vi "Build Log Path.vi"(11 "Project Path":path) -> (0 "error out":errorcluster, 3 "PantherLAB Log File Path":path)   [LabVIEW 2016, in "PantherLAB_Scripting.lvlib"]
uses:
  PantherLAB_Scripting.lvlib
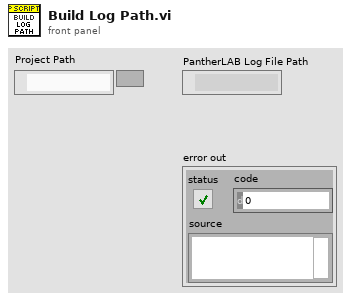
[diagram p1: front panel]
types:
  T1 = enum16{"open", "replace", "create", "open or create", "replace or create", "replace or create with confirmation"}
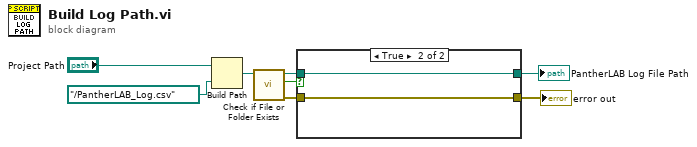
[diagram p0: block diagram]
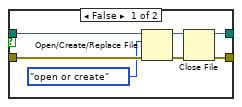
[diagram p2: hidden frame]
diagram:
  n1 = Build Path(base path="Project Path", name or relative path=path "../PantherLAB_Log.csv") -> (appended path=w4:path)
  n2 = call <vilib>:"Check if File or Folder Exists.vi"("path"=w4) -> ("error out"=w8:errorcluster, "file or folder exists?"=w3:bool, "dup path"=w2:path)  [unwired: 8 in]
  n3 = case shown="True" w3 {
    tunnel: w2 -> [w12 w17]
    tunnel: [w9 w17] -> w1
    tunnel: [w14 w16] -> w7
    tunnel: w8 -> [w13 w16]
    frame False {
      n4 = Open/Create/Replace File(file path (use dialog)=w12, error in=w13, operation (0:open)=T1."open or create") -> (refnum out=w10:refnum<file>, error out=w15:errorcluster)  [unwired: 3 in, 1 out]
      n5 = Close File(refnum=w10, error in=w15) -> (path=w9:path, error out=w14:errorcluster)
    }
    frame True {
    }
  }
  "PantherLAB Log File Path" <- w1
  "error out" <- w7
